vi "Write Limit Volt.vi"(8 "error in":errorcluster, 10 "OverVoltage_Protect":dbl, 11 "79XRP in":refnum<class "7976A.lvclass">) -> (0 "error out":errorcluster, 3 "79XRP out":refnum<class "7976A.lvclass">)   [LabVIEW 2019, in "7976A.lvlib" / "7976A.lvclass"]
uses:
  Library/7976A.lvclass
  builds/Instruments/PowerSupply.lvlibp/Library/PowerSupply.lvclass
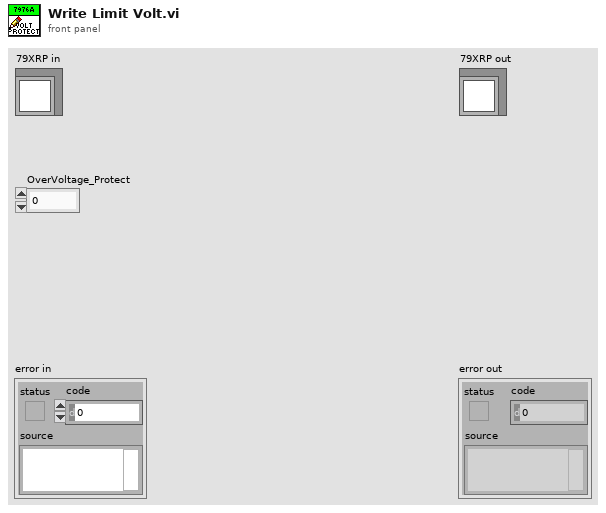
[diagram p1: front panel]
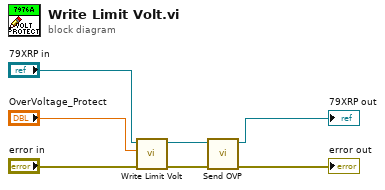
[diagram p0: block diagram]
diagram:
  n1 = call-parent "Write Limit Volt.vi"("error in"="error in", "OverVoltage_Protect"="OverVoltage_Protect", "PowerSupply in"="79XRP in") -> ("error out"=w3:errorcluster, "PowerSupply out"=w4:refnum<class "7976A.lvclass">)  [unwired: 7 in]
  n2 = call "Send OVP.vi"("error in (no error)"=w3, "79XRP in"=w4) -> ("error out"=→"error out":errorcluster, "79XRP out"=→"79XRP out":refnum<class "7976A.lvclass">)  [unwired: 8 in]
